vi "Create or empty folder.vi"(8 "error in (no error)":errorcluster, 9 "Trial Number":i32, 10 "name of folder to create or empty":string, 11 "Experiment folder path":path) -> (0 "error out":errorcluster, 3 "appended path":path)   [LabVIEW 2020]
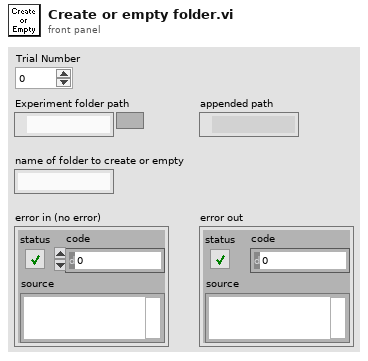
[diagram p1: front panel]
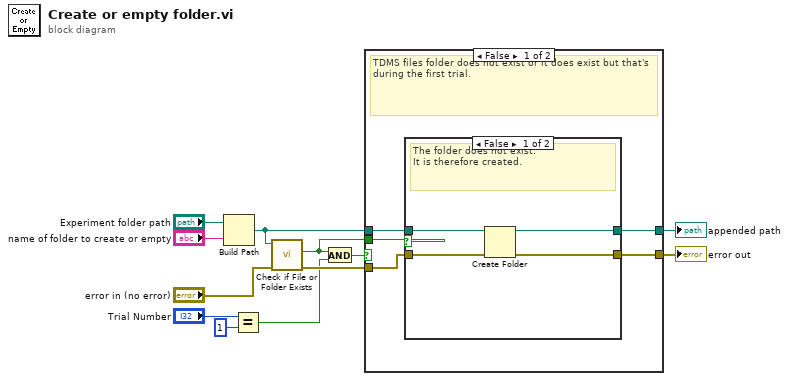
[diagram p0: block diagram]
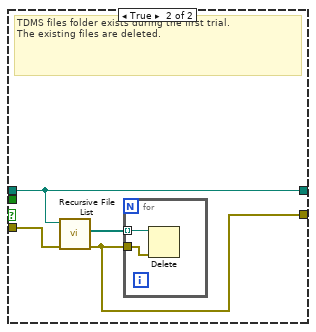
[diagram p3: hidden frame]
diagram:
  n1 = Build Path(base path="Experiment folder path", name or relative path="name of folder to create or empty") -> (appended path=w10:path)
  n2 = Equal?(x="Trial Number", y=1) -> (x = y?=w3:bool)
  n3 = call <vilib>:"Check if File or Folder Exists.vi"("error in (no error)"="error in (no error)", "path"=w10) -> ("error out"=w12:errorcluster, "file or folder exists?"=w1:bool)  [unwired: 7 in, 1 out]
  n4 = And(x=w1, y=w3) -> (x .and. y?=w2:bool)
  n5 = case shown="False" w2 {
    tunnel: [w17 w27] -> w8
    tunnel: [w16 w24] -> w9
    tunnel: w10 -> [w15 w27]
    tunnel: w12 -> [w14 w25]
    tunnel: w1 -> [w13 _]
    frame False {
      # "TDMS files folder does not exist or it does exist but that's during the first trial."
      n6 = case shown="False" w13 {
        tunnel: [w21 w23] -> w17
        tunnel: [w20 w22] -> w16
        tunnel: w15 -> [w19 w23]
        tunnel: w14 -> [w18 w22]
        frame False {
          # "The folder does not exist.\nIt is therefore created."
          n7 = Create Folder(path (use dialog)=w19, error in=w18) -> (created path=w21:path, error out=w20:errorcluster)  [unwired: 1 in, 1 out]
        }
        frame True {
          # "Folder exists but that's expected as this is not the first trial"
        }
      }
    }
    frame True {
      # "TDMS files folder exists during the first trial.\nThe existing files are deleted."
      n8 = call <vilib>:"Recursive File List.vi"("error in (no error)"=w25, "Folder Path"=w27) -> ("error out"=w24:errorcluster, "All Files in Dir"=w26:path[])  [unwired: 5 in, 3 out]
      n9 = for {
        tunnel: w26 -> [w29] mode=indexing
        tunnel: w24 -> [w28]
        n10 = Delete(path (use dialog)=w29, error in=w28) -> ()  [unwired: 3 in, 3 out]
      }
    }
  }
  "error out" <- w9
  "appended path" <- w8
